vi "create_full_token.vi"(8 "error in (no error)":errorcluster, 11 "llm_azureopenai_chatmodels in":refnum<class "llm_azureopenai_chatmodels.lvclass">) -> (0 "error out":errorcluster, 1 "token":string, 2 "header":string(combo)="Authorization", 3 "llm_azureopenai_chatmodels out":refnum<class "llm_azureopenai_chatmodels.lvclass">)   [LabVIEW 2020, in "llm_azureopenai_chatmodels.lvclass"]
uses:
  llm_azureopenai_chatmodels.lvclass
  D:/Personal/LabVIEW LLMs/src/models/llm_openai_chatmodels/llm_openai_chatmodels.lvclass
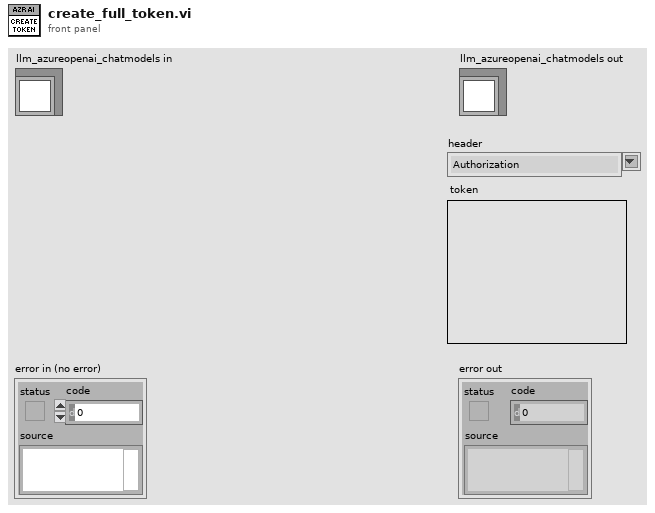
[diagram p1: front panel]
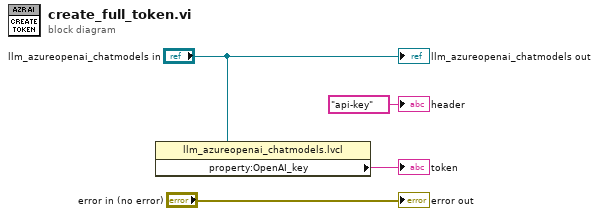
[diagram p0: block diagram]
diagram:
  n1 = property class="llm_azureopenai_chatmodels.lvcl"(reference="llm_azureopenai_chatmodels in") -> ("property:OpenAI_key"=→"token":string)  [unwired: 1 in, 2 out]
  "error out" <- "error in (no error)"
  "llm_azureopenai_chatmodels out" <- "llm_azureopenai_chatmodels in"
  "header" <- "api-key" ("header")
